vi "Diagnostics.CheckTimeout.vi"(8 "error in (no error)":errorcluster) -> (0 "error out":errorcluster, 3 "Timeout":bool)   [LabVIEW 2024, in "Diagnostics Addon Engine.lvlib"]
uses:
  Diagnostics Addon Engine.lvlib
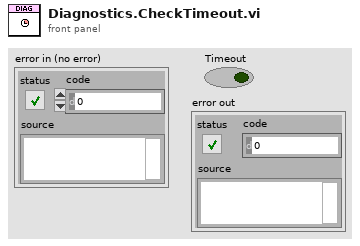
[diagram p1: front panel]
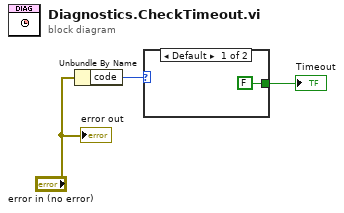
[diagram p0: block diagram]
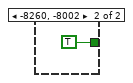
[diagram p2: hidden frame]
diagram:
  n1 = Unbundle By Name("error in (no error)") -> ("code"=w2:i32)
  n2 = case shown="Default" w2 {
    tunnel: [FALSE TRUE] -> w3
    frame Default {
    }
    frame -8260, -8002 {
    }
  }
  "Timeout" <- w3
  "error out" <- "error in (no error)"
